vi "Roots_2_poly.vi"(8 "error in (no error)":errorcluster, 11 "Roots":cdb[](array[numeric])) -> (0 "error out":errorcluster, 3 "Polynomial Coeffcients":dbl[](array[numeric]))   [LabVIEW 2020, in "PC-RT_Controller.lvlib"]
doc: "Convert roots into polynomial coefficients. Used to convert ZPK to TF."
uses:
  PC-RT_Controller.lvlib
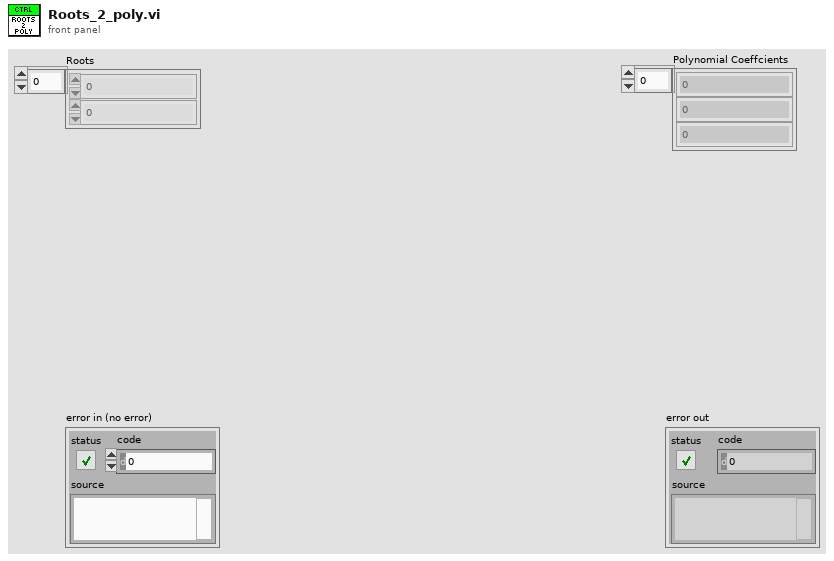
[diagram p1: front panel]
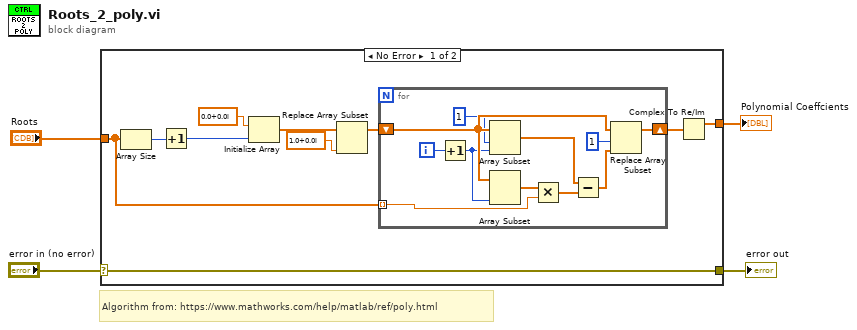
[diagram p0: block diagram]
diagram:
  # "Algorithm from: https://www.mathworks.com/help/matlab/ref/poly.html"
  n1 = case shown="No Error" "error in (no error)" {
    selector: "error in (no error)" -> [w14 w26]
    tunnel: [w14 w26] -> w3
    tunnel: "Roots" -> [w7 _]
    tunnel: [w5 _] -> w1
    frame No Error {
      n2 = Array Size(array=w7) -> (size(s)=w9:i32)
      n3 = Increment(x=w9) -> (x+1=w8:i32)
      n4 = Initialize Array(cdb 0.0+0.0i ("element"), w8) -> (w12:cdb[])
      n5 = Replace Array Subset(array=w12, new element=cdb 1.0+0.0i ("new element/subarray")) -> (w10:cdb[])  [unwired: 1 in]
      n6 = for {
        tunnel: w7 -> [w23] mode=indexing
        shift-right: [w25] -> w6
        shift-left: w10 -> [w22]
        i -> [w20]
        n7 = Increment(x=w20) -> (x+1=w15:i32)
        n8 = Array Subset(array=w22, index=1, length=w15) -> (w19:cdb[])
        n9 = Array Subset(array=w22, length=w15) -> (w24:cdb[])  [unwired: 1 in]
        n10 = Multiply(x=w24, y=w23) -> (x*y=w18:cdb[])
        n11 = Subtract(x=w19, y=w18) -> (x-y=w17:cdb[])
        n12 = Replace Array Subset(array=w22, new element=w17, index=1) -> (w25:cdb[])
      }
      n13 = Complex To Re/Im(x + iy=w6) -> (x=w5:dbl[])  [unwired: 1 out]
    }
    frame Error {
    }
  }
  "error out" <- w3
  "Polynomial Coeffcients" <- w1
